vi "SetLaserPower.vi"(8 "error in":errorcluster, 9 "AOTF3":dbl, 10 "AOTF2":dbl, 11 "AOTF1":dbl) -> (0 "error out":errorcluster)   [LabVIEW 2015]
uses:
  <vilib>/DAQmx/write.llb/DAQmx Write.vi
  <vilib>/DAQmx/write.llb/DAQmx Write (Analog 1D DBL NChan 1Samp).vi
  <vilib>/DAQmx/miscellaneous.llb/DAQmx Fill In Error Info.vi
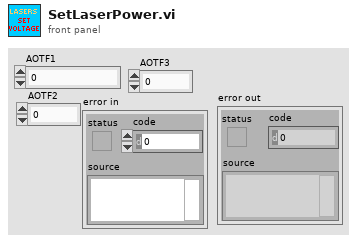
[diagram p1: front panel]
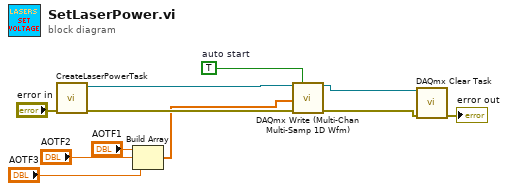
[diagram p0: block diagram]
diagram:
  w11 = TRUE  # auto start
  n1 = call "CreateLaserPowerTask.vi"("error in"="error in") -> ("error out"=w9:errorcluster, "task out"=w10:refnum<k21>)  [unwired: 9 in]
  n2 = Build Array("AOTF1", "AOTF2", "AOTF3") -> (w5:dbl[])
  n3 = call-poly "DAQmx Write (Multi-Chan Multi-Samp 1D Wfm).vi"("task/channels in"=w10, "auto start"=w11, "data"=w5, "error in"=w9) -> ("task out"=w4:refnum<k21>, "error out"=w3:errorcluster)  [unwired: 9 in, 1 out]
  n4 = call <vilib>:"DAQmx Clear Task.vi"("task in"=w4, "error in"=w3) -> ("error out"=→"error out":errorcluster)  [unwired: 13 in]
